vi "Configure Channel Coupling Mode.vi"(8 "error in":errorcluster, 10 "coupling mode":u32(ring) items=["API429_CHANNEL_COUPLING_EXT", "API429_CHANNEL_COUPLING_DUAL", "API429_CHANNEL_COUPLING_INT"], 11 "board handle":u8) -> (0 "error out":errorcluster, 3 "board handle out":u8)   [LabVIEW 2024, in "AIM ARINC 429 Hardware API.lvlib"]
uses:
  AIM ARINC 429 Hardware API.lvlib
  <instrlib>/AIM GmbH/_ARINC-429/subvi/Error Converter (ErrCode or Status).vi
  <instrlib>/AIM GmbH/_ARINC-429/subvi/Get Library Path.vi
  <instrlib>/AIM GmbH/_ARINC-429/VIs/Library/Api429Lib Error Desc Get.vi
  <instrlib>/AIM GmbH/_ARINC-429/subvi/Get Error Number Offset.vi
  <vilib>/Utility/error.llb/Error Cluster From Error Code.vi
  <instrlib>/AIM GmbH/_ARINC-429/AIM429LV.lvlib
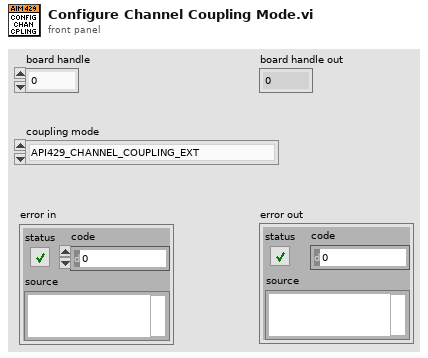
[diagram p1: front panel]
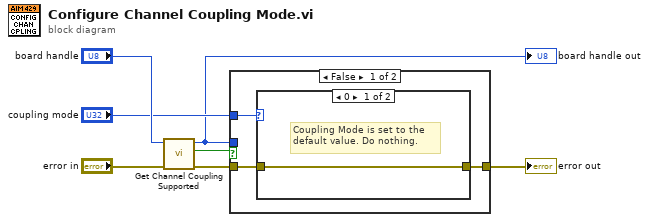
[diagram p0: block diagram]
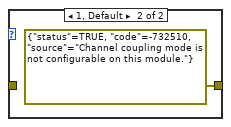
[diagram p2: hidden frame]
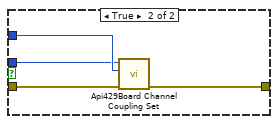
[diagram p3: hidden frame]
diagram:
  n1 = call "Get Channel Coupling Supported.vi"("error in (no error)"="error in", "board_handle"="board handle") -> ("error out"=w2:errorcluster, "Is supported"=w1:bool, "board_handle out"=w4:u8)  [unwired: 7 in]
  "board handle out" <- w4
  n2 = case shown="False" w1 {
    tunnel: w2 -> [w9 w16]
    tunnel: "coupling mode" -> [w8 w15]
    tunnel: w4 -> [_ w14]
    tunnel: [w10 w13] -> w3
    frame False {
      n3 = case shown="0" w8 {
        tunnel: [w11 errorcluster {"status"=TRUE, "code"=-732510, "source"="Channel coupling mode is not configurable on this module."} ("error out")] -> w10
        tunnel: w9 -> [w11 _]
        frame 0 {
          # "Coupling Mode is set to the\ndefault value. Do nothing."
        }
        frame 1, Default {
        }
      }
    }
    frame True {
      n4 = call <instrlib>:"Api429Board Channel Coupling Set.vi"("error in (no error)"=w16, "coupling"=w15, "board_handle"=w14) -> ("error out"=w13:errorcluster)  [unwired: 8 in]
    }
  }
  "error out" <- w3
